vi "Get Columns.vi"(0 "Device in":refnum<class "Device.lvclass">, 1 "error in (no error)":errorcluster) -> (2 "Device out":refnum<class "Device.lvclass">, 3 "Columns":refnum<class "Column.lvclass">[](array[class]), 4 "error out":errorcluster)   [LabVIEW 2013, in "Device.lvclass"]
uses:
  Device.lvclass
  ColumnVIs/Column/Column.lvclass
  Device.lvclass/Device.ctl
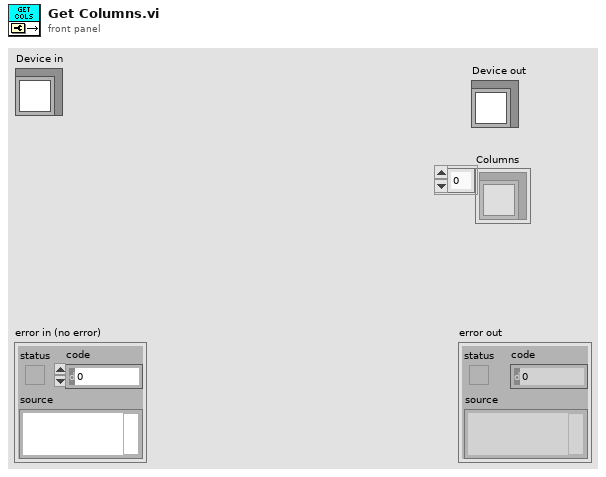
[diagram p1: front panel]
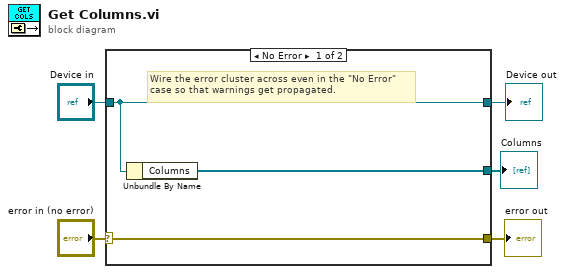
[diagram p0: block diagram]
diagram:
  n1 = case shown="No Error" "error in (no error)" {
    selector: "error in (no error)" -> [w8 w10]
    tunnel: [w8 w10] -> w4
    tunnel: [w7 w9] -> w2
    tunnel: "Device in" -> [w7 w9]
    tunnel: [w6 _] -> w1
    frame No Error {
      # "Wire the error cluster across even in the \"No Error\"\ncase so that warnings get propagated."
      n2 = Unbundle By Name(w7) -> ("Columns"=w6:refnum<class "Column.lvclass">[])
    }
    frame Error {
    }
  }
  "error out" <- w4
  "Device out" <- w2
  "Columns" <- w1
